vi "ViHandler.CheckForExistingVi.Main.vi"(8 "ErrorIn":errorcluster, 10 "ViQueueName":string, 11 "ViReference":refnum<vi>) -> (0 "ErrorOut":errorcluster, 2 "Found?":bool, 3 "ViInfo":T1)   [LabVIEW 2016, in "ViHandler.lvclass"]
uses:
  ViHandler.lvclass
  ViHandler.ViInfo.ctl
  ObjectHandler/ObjectHandler.GetObjectWType.ctl
  ObjectHandler/ObjectHandler.ObjectWType.ctl
  ObjectHandler/ObjectHandler.ObjectType.ctl
  ObjectHandler/ObjectHandler.lvclass
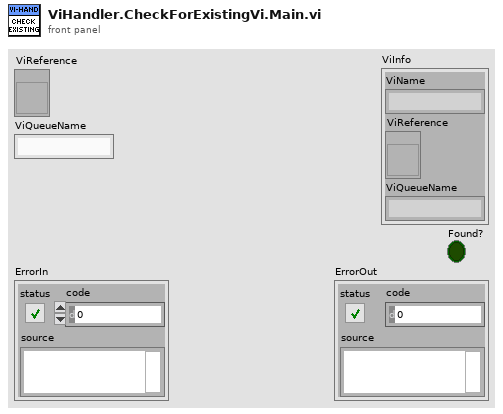
[diagram p1: front panel]
types:
  T1 = typedef "ViHandler.lvclass/ViHandler.ViInfo.ctl" = cluster{"ViName":string, "ViReference":refnum<vi>, "ViQueueName":string}
  T2 = typedef "ObjectHandler.lvclass/ObjectHandler.GetObjectWType.ctl" = cluster{"Name":string, "Caller":string}
  T3 = typedef "ObjectHandler.lvclass/ObjectHandler.ObjectWType.ctl" = cluster{"ObjectType":T4, "Object":variant}
  T4 = typedef "ObjectHandler.lvclass/ObjectHandler.ObjectType.ctl" = enum16{"undefined", "ObjectHandler", "ViHandler", "ErrorHandler", "CentralStorage", "Hausmodell", "Sondenmodell", "Wärmepumpe", "Umgebung"}
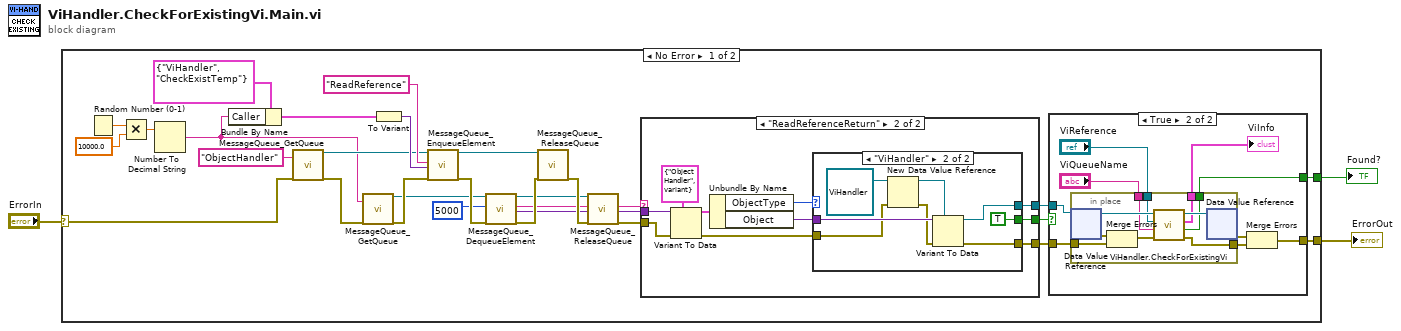
[diagram p0: block diagram]
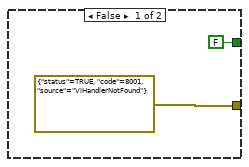
[diagram p2: hidden frame]
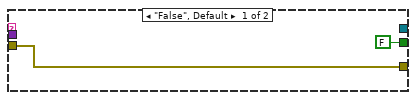
[diagram p3: hidden frame]
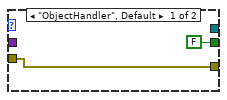
[diagram p4: hidden frame]
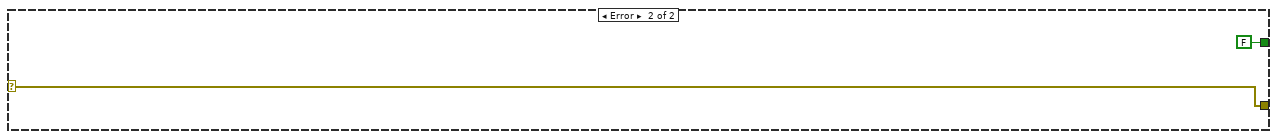
[diagram p5: hidden frame]
diagram:
  n1 = case shown="No Error" "ErrorIn" {
    selector: "ErrorIn" -> [w12 w76]
    tunnel: [w13 w76] -> w3
    tunnel: [w10 FALSE ("Found?")] -> w1
    frame No Error {
      n2 = Random Number (0-1)() -> (number: 0 to 1=w7:dbl)
      n3 = Multiply(x=w7, y=10000.0) -> (x*y=w5:dbl)
      n4 = Number To Decimal String(number=w5) -> (decimal integer string=w4:string)  [unwired: 1 in]
      n5 = Bundle By Name(cluster=T2 {"Name"="ViHandler", "Caller"="CheckExistTemp"} ("GetRefInput"), "Caller"=w4) -> (w8:T2)
      n6 = call "MessageQueue_GetQueue.vi"("Name"="ObjectHandler", "ErrorIn"=w12) -> ("QueueOut"=w17:refnum<queue>, "ErrorOut"=w18:errorcluster)  [unwired: 15 in, 1 out]
      n7 = call "MessageQueue_GetQueue.vi"("Name"=w4, "ErrorIn"=w18) -> ("QueueOut"=w23:refnum<queue>, "ErrorOut"=w26:errorcluster)  [unwired: 15 in, 1 out]
      n8 = To Variant(anything=w8) -> (Variant=w27:variant)
      n9 = call "MessageQueue_EnqueueElement.vi"("QueueIn"=w17, "Message"="ReadReference", "Data"=w27, "ErrorIn"=w26) -> ("QueueOut"=w20:refnum<queue>, "ErrorOut"=w25:errorcluster)  [unwired: 14 in]
      n10 = call "MessageQueue_DequeueElement.vi"("QueueIn"=w23, "Timeout"=5000, "ErrorIn"=w25) -> ("QueueOut"=w19:refnum<queue>, "Message"=w22:string, "Data"=w21:variant, "ErrorOut"=w31:errorcluster)  [unwired: 12 in, 1 out]
      n11 = call "MessageQueue_ReleaseQueue.vi"("QueueIn"=w20, "ErrorIn"=w31) -> ("ErrorOut"=w30:errorcluster)  [unwired: 15 in, 2 out]
      n12 = call "MessageQueue_ReleaseQueue.vi"("QueueIn"=w19, "ErrorIn"=w30) -> ("ErrorOut"=w16:errorcluster)  [unwired: 15 in, 2 out]
      n13 = case shown="\"ReadReferenceReturn\"" w22 {
        tunnel: w21 -> [_ w64]
        tunnel: [w53 w60] -> w15
        tunnel: w16 -> [w53 w58]
        tunnel: [FALSE w56] -> w14
        tunnel: [_ w55] -> w11
        frame "False", Default {
        }
        frame "ReadReferenceReturn" {
          n14 = Variant To Data(error in=w58, type=T3 {"ObjectType"=enum."ObjectHandler", "Object"=variant} ("ObjectWType"), Variant=w64) -> (data=w63:T3, error out=w57:errorcluster)
          n15 = Unbundle By Name(w63) -> ("ObjectType"=w62:T4, "Object"=w61:variant)
          n16 = case shown="\"ViHandler\"" w62 {
            tunnel: w61 -> [_ w74]
            tunnel: [w65 w71] -> w60
            tunnel: w57 -> [w65 w70]
            tunnel: [FALSE TRUE] -> w56
            tunnel: [_ w67] -> w55
            frame "ObjectHandler", Default {
            }
            frame "ViHandler" {
              n17 = New Data Value Reference(data value=refnum<class "ViHandler.lvclass"> refnum ("ViHandler.lvclass"), error in=w70) -> (data value reference=w72:refnum<data-value>, error out=w69:errorcluster)
              n18 = Variant To Data(error in=w69, type=w72, Variant=w74) -> (data=w67:refnum<data-value>, error out=w71:errorcluster)
            }
          }
        }
      }
      n19 = case shown="True" w14 {
        tunnel: w15 -> [_ w40]
        tunnel: [errorcluster {"status"=TRUE, "code"=8001, "source"="ViHandlerNotFound"} ("error IO") w39] -> w13
        tunnel: w11 -> [_ w35]
        tunnel: [FALSE ("Found?") w34] -> w10
        frame False {
        }
        frame True {
          n20 = in-place {
            in-place-border: [w50] -> w42
            in-place-border: w40 -> [w51]
            in-place-border: [w46] -> w38
            in-place-border: [w45] -> w34
            in-place-border: "ViReference" -> [w44]
            in-place-border: "ViQueueName" -> [w43]
            n21 = in-place-dvr #1(w35) -> (w48:refnum<class "ViHandler.lvclass">, w52:errorcluster)
            n22 = Merge Errors(w52, w51) -> (w49:errorcluster)
            n23 = call "ViHandler.CheckForExistingVi.vi"("error in (no error)"=w49, "ViQueueName"=w43, "ViReference"=w44, "ViHandler in"=w48) -> ("error out"=w50:errorcluster, "Found?"=w45:bool, "ViInfo"=w46:T1, "ViHandler out"=w47:refnum<class "ViHandler.lvclass">)  [unwired: 4 in]
            n24 = in-place-dvr #1(w47) -> (w41:errorcluster)  [unwired: 1 out]
          }
          "ViInfo" <- w38
          n25 = Merge Errors(w41, w42) -> (w39:errorcluster)
        }
      }
    }
    frame Error {
    }
  }
  "ErrorOut" <- w3
  "Found?" <- w1
